vi "TestLines.vi"() -> ()   [LabVIEW 2012]
doc: "A VI for debugging math errors in the linear interpreter."
panel:
  in  "Angles":dbl[](array[numeric])
  in  "Values":dbl[](array[numeric])
  out "Intercept":dbl[](array[numeric])
  out "Slope":dbl[](array[numeric])
  out "Angles/Indicies":dbl[](array[numeric])
  in  "Desired Angle Input":dbl
  out "Value Output":dbl
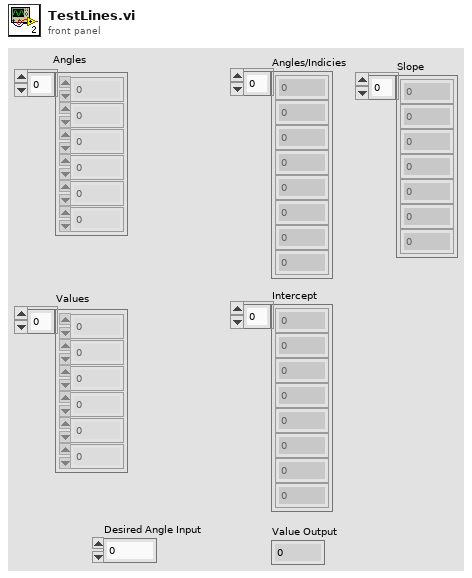
[diagram p1: front panel]
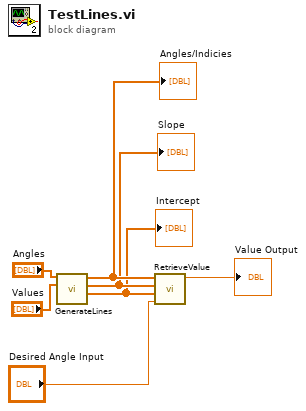
[diagram p0: block diagram]
diagram:
  n1 = call "GenerateLines.vi"("Values"="Values", "Angles"="Angles") -> ("Intercept"=w3:dbl[], "Slope"=w4:dbl[], "Angles/Indicies"=w5:dbl[])  [unwired: 7 in]
  "Angles/Indicies" <- w5
  "Slope" <- w4
  "Intercept" <- w3
  n2 = call "RetrieveValue.vi"("Desired Angle Input"="Desired Angle Input", "Intercept"=w3, "Slope"=w4, "Angles/Indicies"=w5) -> ("Value Output"=→"Value Output":dbl)  [unwired: 7 in]
